vi "Write value.vi"(8 "error in (no error)":errorcluster, 10 "Value":i32, 11 "Ring D Element in":refnum<class "String dropdown D Element.lvclass">) -> (0 "error out":errorcluster, 3 "Ring D Element out":refnum<class "String dropdown D Element.lvclass">)   [LabVIEW 2018, in "D Datagrid Library.lvlib" / "String dropdown D Element.lvclass"]
uses:
  String dropdown D Element.lvclass
  String dropdown D Element.lvclass/String dropdown D Element.ctl
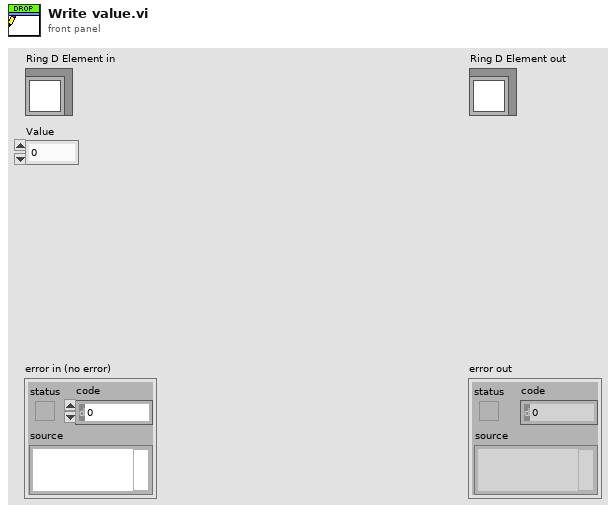
[diagram p1: front panel]
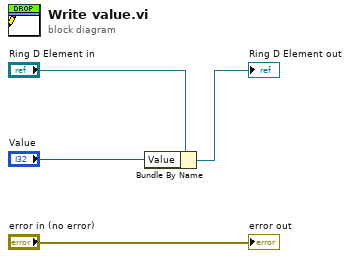
[diagram p0: block diagram]
diagram:
  n1 = Bundle By Name(cluster="Ring D Element in", "Value"="Value") -> (→"Ring D Element out":refnum<class "String dropdown D Element.lvclass">)
  "error out" <- "error in (no error)"
